vi "Close Document anf PDFWriter.vi"(0 "PDF Report IN":refnum<class "PDF Report Class.lvclass">, 11 "error in (no error)":errorcluster) -> (4 "PDF Report OUT":refnum<class "PDF Report Class.lvclass">, 15 "error out":errorcluster)   [LabVIEW 2019]
doc: "Version 1.0\nDeveloped by Jean-Marc Simard\nCopyright © 2010, Exaprom Inc.\nAll rights reserved.\nLicense: BSD\n\nWith iTextSharp 4.1.6 (http://itextsharp.sourceforge.net)\nunder Mozilla Public License Version 1.1\n(http://www.mozilla.org/MPL/MPL-1.1.html)"
uses:
  <userlib>/Exaprom PDF/LV Class/PDF Report Class/PDF Report Class.lvclass
  C:/Program Files/National Instruments/LabVIEW 2019/user.lib/Exaprom PDF/DLL/itextsharp.dll
  DLL/itextsharp.dll
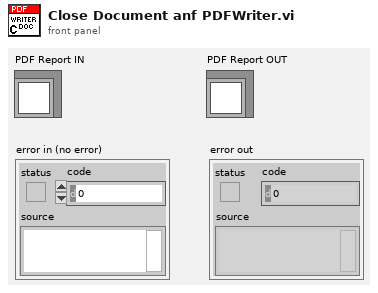
[diagram p1: front panel]
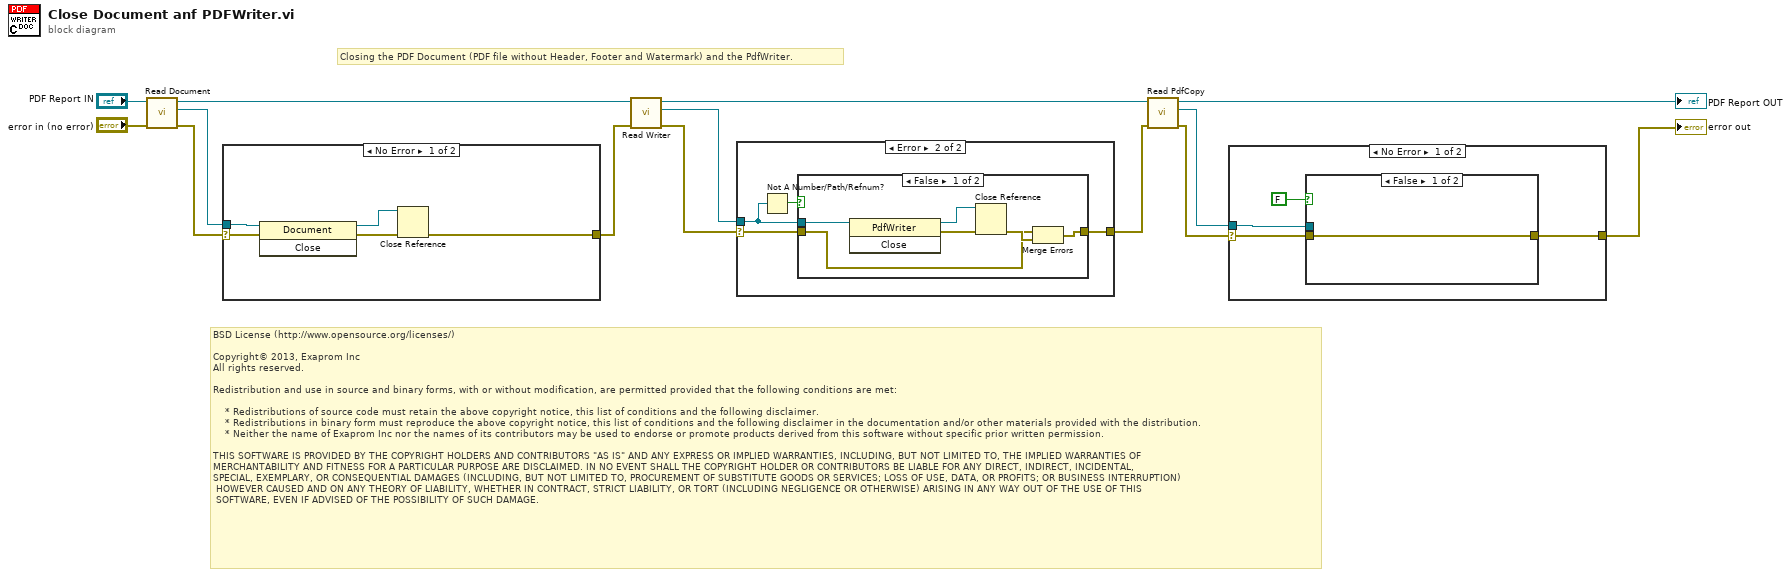
[diagram p0: block diagram]
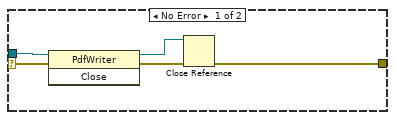
[diagram p2: hidden frame]
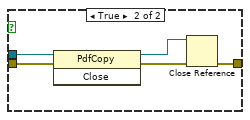
[diagram p4: hidden frame]
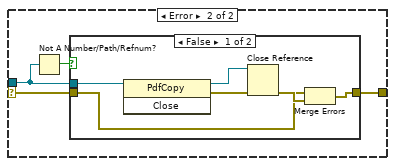
[diagram p5: hidden frame]
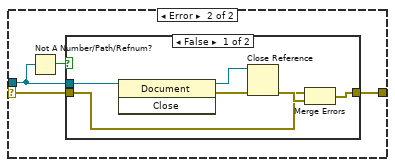
[diagram p7: hidden frame]
diagram:
  # "Closing the PDF Document (PDF file without Header, Footer and Watermark) and the PdfWriter."
  # "BSD License (http://www.opensource.org/licenses/)\n\nCopyright© 2013, Exaprom Inc\nAll rights reserved.\n\nRedistribution and use in source and binary forms, with or without modification, are permitted provided that the following conditions are met:\n\n    * Redistributions of source code must retain the above copyright notice, this list of conditions and the following disclaimer.\n    * Redistributions in binary form must reproduce the above copyright notice, this list of conditions and the following disclaimer in the documentation and/or other materials provided with the distribution.\n    * Neither the name of Exaprom Inc nor the names of its contributors may be used to endorse or promote products derived from this software without specific prior written permission.\n\nTHIS SOFTWARE IS PROVIDED BY THE COPYRIGHT HOLDERS AND CONTRIBUTORS \"AS IS\" AND ANY EXPRESS OR IMPLIED WARRANTIES, INCLUDING, BUT NOT LIMITED TO, THE IMPLIED WARRANTIES OF \nMERCHANTABILITY AND FITNESS FOR A PARTICULAR PURPOSE ARE DISCLAIMED. IN NO EVENT SHALL THE COPYRIGHT HOLDER OR CONTRIBUTORS BE LIABLE FOR ANY DIRECT, INDIRECT, INCIDENTAL,\nSPECIAL, EXEMPLARY, OR CONSEQUENTIAL DAMAGES (INCLUDING, BUT NOT LIMITED TO, PROCUREMENT OF SUBSTITUTE GOODS OR SERVICES; LOSS OF USE, DATA, OR PROFITS; OR BUSINESS INTERRUPTION)\n HOWEVER CAUSED AND ON ANY THEORY OF LIABILITY, WHETHER IN CONTRACT, STRICT LIABILITY, OR TORT (INCLUDING NEGLIGENCE OR OTHERWISE) ARISING IN ANY WAY OUT OF THE USE OF THIS\n SOFTWARE, EVEN IF ADVISED OF THE POSSIBILITY OF SUCH DAMAGE."
  n1 = call-dynamic "Read Document.vi"("error in (no error)"="error in (no error)", "PDF Report Class in"="PDF Report IN") -> ("error out"=w9:errorcluster, "Document"=w11:refnum<k24>, "PDF Report Class out"=w13:refnum<class "PDF Report Class.lvclass">)  [unwired: 7 in]
  n2 = case shown="No Error" w9 {
    selector: w9 -> [w16 w22]
    tunnel: [w18 w23] -> w8
    tunnel: w11 -> [w15 w21]
    frame No Error {
      n3 = invoke class="Document" method="Close"(reference=w15, error in=w16) -> (reference out=w19:refnum<k24>, error out=w17:errorcluster)  [unwired: 1 in, 1 out]
      n4 = Close Reference(reference=w19, error in (no error)=w17) -> (error out=w18:errorcluster)
    }
    frame Error {
      n5 = Not A Number/Path/Refnum?(number/path/refnum=w21) -> (NaN/Path/Refnum?=w20:bool)
      n6 = case shown="False" w20 {
        tunnel: [w24 w30] -> w23
        tunnel: w22 -> [w25 w30]
        tunnel: w21 -> [w27 _]
        frame False {
          n7 = invoke class="Document" method="Close"(reference=w27) -> (reference out=w29:refnum<k24>, error out=w28:errorcluster)  [unwired: 2 in, 1 out]
          n8 = Close Reference(reference=w29, error in (no error)=w28) -> (error out=w26:errorcluster)
          n9 = Merge Errors(w25, w26) -> (w24:errorcluster)
        }
        frame True {
        }
      }
    }
  }
  n10 = call-dynamic "Read Writer.vi"("error in (no error)"=w8, "PDF Report Class in"=w13) -> ("error out"=w2:errorcluster, "Writer"=w1:refnum<k24>, "PDF Report Class out"=w12:refnum<class "PDF Report Class.lvclass">)  [unwired: 7 in]
  n11 = case shown="Error" w2 {
    selector: w2 -> [w32 w38]
    tunnel: [w34 w39] -> w3
    tunnel: w1 -> [w31 w37]
    frame No Error {
      n12 = invoke class="PdfWriter" method="Close"(reference=w31, error in=w32) -> (reference out=w35:refnum<k24>, error out=w33:errorcluster)  [unwired: 1 in, 1 out]
      n13 = Close Reference(reference=w35, error in (no error)=w33) -> (error out=w34:errorcluster)
    }
    frame Error {
      n14 = Not A Number/Path/Refnum?(number/path/refnum=w37) -> (NaN/Path/Refnum?=w36:bool)
      n15 = case shown="False" w36 {
        tunnel: [w40 w46] -> w39
        tunnel: w38 -> [w41 w46]
        tunnel: w37 -> [w43 _]
        frame False {
          n16 = invoke class="PdfWriter" method="Close"(reference=w43) -> (reference out=w45:refnum<k24>, error out=w44:errorcluster)  [unwired: 2 in, 1 out]
          n17 = Close Reference(reference=w45, error in (no error)=w44) -> (error out=w42:errorcluster)
          n18 = Merge Errors(w41, w42) -> (w40:errorcluster)
        }
        frame True {
        }
      }
    }
  }
  n19 = call-dynamic "Read PdfCopy.vi"("error in (no error)"=w3, "PDF Report Class in"=w12) -> ("error out"=w6:errorcluster, "PdfCopy"=w5:refnum<k24>, "PDF Report Class out"=→"PDF Report OUT":refnum<class "PDF Report Class.lvclass">)  [unwired: 7 in]
  n20 = case shown="No Error" w6 {
    selector: w6 -> [w49 w59]
    tunnel: [w50 w60] -> w4
    tunnel: w5 -> [w48 w58]
    frame No Error {
      n21 = case shown="False" FALSE {
        tunnel: [w51 w55] -> w50
        tunnel: w49 -> [w51 w53]
        tunnel: w48 -> [_ w52]
        frame False {
        }
        frame True {
          n22 = invoke class="PdfCopy" method="Close"(reference=w52, error in=w53) -> (reference out=w56:refnum<k24>, error out=w54:errorcluster)  [unwired: 1 in, 1 out]
          n23 = Close Reference(reference=w56, error in (no error)=w54) -> (error out=w55:errorcluster)
        }
      }
    }
    frame Error {
      n24 = Not A Number/Path/Refnum?(number/path/refnum=w58) -> (NaN/Path/Refnum?=w57:bool)
      n25 = case shown="False" w57 {
        tunnel: [w61 w67] -> w60
        tunnel: w59 -> [w62 w67]
        tunnel: w58 -> [w64 _]
        frame False {
          n26 = invoke class="PdfCopy" method="Close"(reference=w64) -> (reference out=w66:refnum<k24>, error out=w65:errorcluster)  [unwired: 2 in, 1 out]
          n27 = Close Reference(reference=w66, error in (no error)=w65) -> (error out=w63:errorcluster)
          n28 = Merge Errors(w62, w63) -> (w61:errorcluster)
        }
        frame True {
        }
      }
    }
  }
  "error out" <- w4
